vi "lv_buzzer.vi"() -> ()   [LabVIEW 2016]
panel:
  in  "Slide":dbl(slide) scale=0.0..10.0
  in  "Boolean 12":bool
  in  "Boolean 11":bool
  in  "Boolean 9":bool
  in  "Boolean 6":bool
  out "Numeric 4":dbl caption="Strange"
  out "Boolean 10":bool caption="Strange"
  out "text":string
  out "Boolean 8":bool
  out "Boolean 7":bool
  in  "file path (use dialog)":path
  in  "Boolean 5":bool
  in  "Boolean 4":bool
  out "Numeric 3":dbl caption="Down"
  out "Numeric 2":dbl caption="Up"
  out "Charm":dbl
  out "Boolean 3":bool caption="Down"
  out "Boolean 2":bool caption="Up"
  out "Boolean":bool caption="Charm"
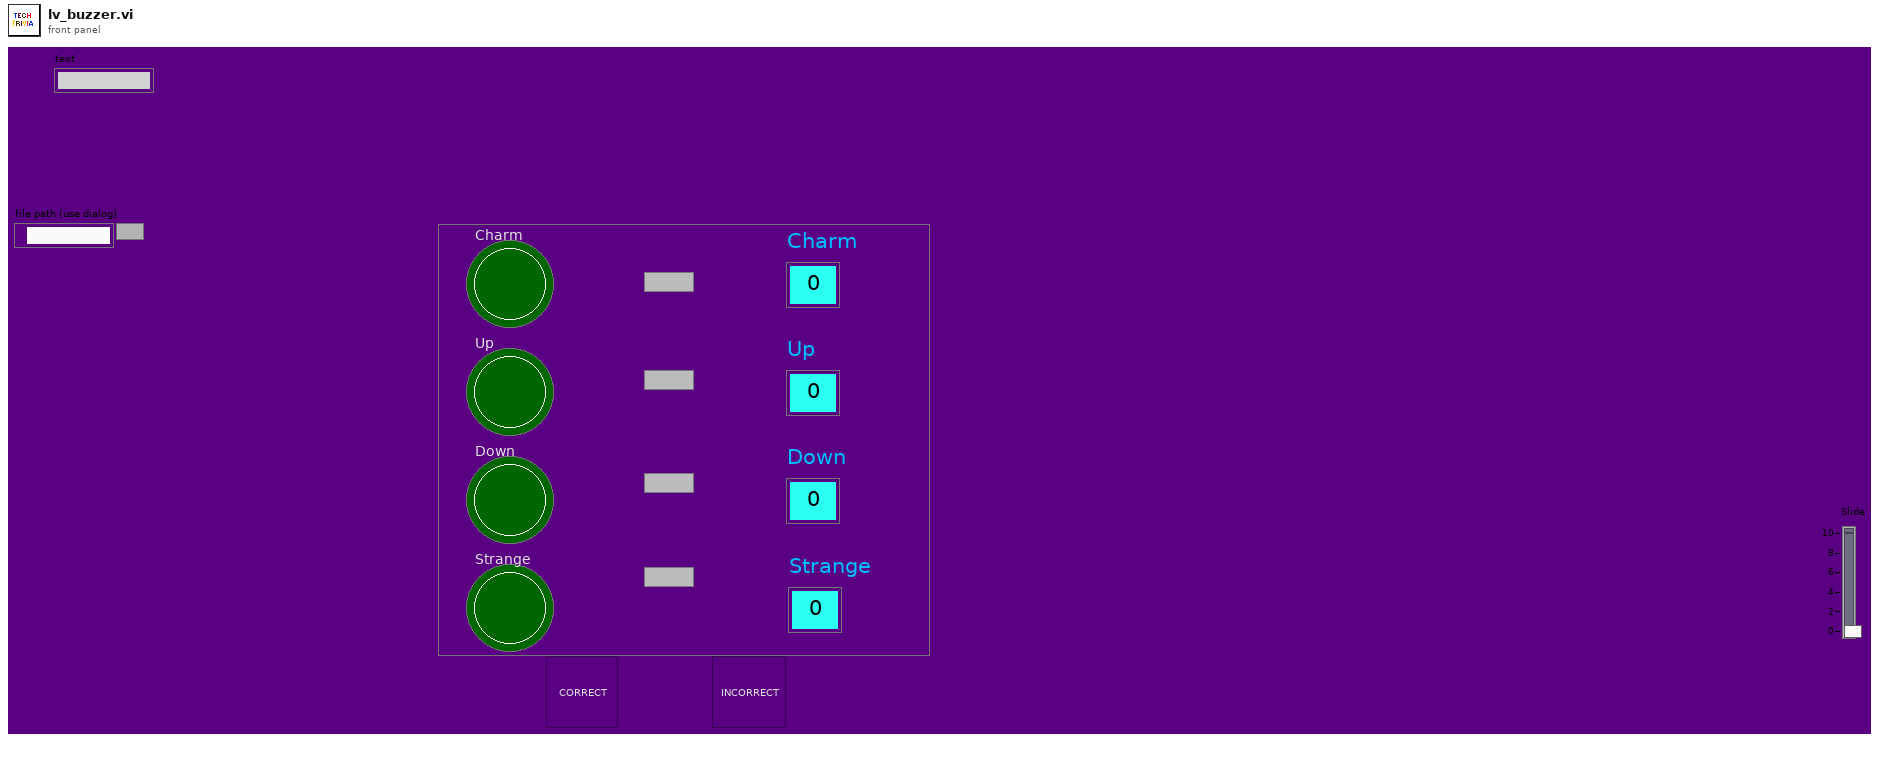
[diagram p1: front panel]
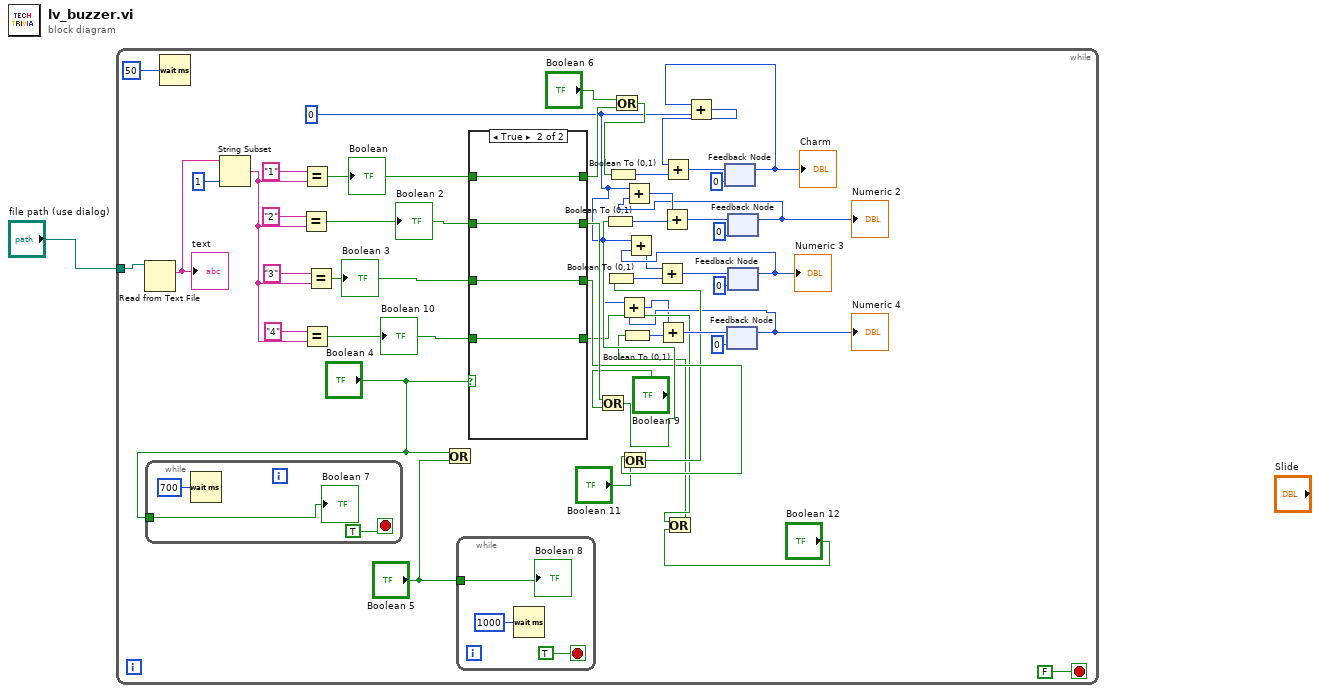
[diagram p0: block diagram]
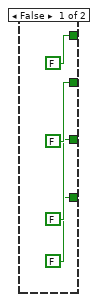
[diagram p2: hidden frame]
diagram:
  n1 = while {
    tunnel: "file path (use dialog)" -> [w32]
    stop <- FALSE stop-if-true
    w4 = i16 0 ("y")
    n2 = Read from Text File(file (use dialog)=w32) -> (text=w38:string)  [unwired: 3 in, 3 out]
    "text" <- w38
    n3 = while {
      tunnel: "Boolean 4" -> [w56]
      stop <- TRUE stop-if-true
      n4 = Wait (ms)(milliseconds to wait=u32 700) -> ()  [unwired: 1 out]
      "Boolean 7" <- w56
    }
    n5 = Wait (ms)(milliseconds to wait=u32 50) -> ()  [unwired: 1 out]
    n6 = String Subset(string=w38, length (rest)=1 ("length (rest)")) -> (substring=w28:string)  [unwired: 1 in]
    n7 = Equal?(x="2", y=w28) -> (x = y?=w30:bool)
    "Boolean 2" <- w30
    n8 = Equal?(x="1", y=w28) -> (x = y?=w31:bool)
    "Boolean" <- w31
    n9 = Equal?(x="4", y=w28) -> (x = y?=w26:bool)
    "Boolean 10" <- w26
    n10 = Equal?(x="3", y=w28) -> (x = y?=w29:bool)
    "Boolean 3" <- w29
    n11 = Or(x="Boolean 4", y="Boolean 5") -> ()  [unwired: 1 out]
    n12 = while {
      tunnel: "Boolean 5" -> [w53]
      stop <- TRUE stop-if-true
      n13 = Wait (ms)(milliseconds to wait=u32 1000) -> ()  [unwired: 1 out]
      "Boolean 8" <- w53
    }
    n14 = case shown="True" "Boolean 4" {
      tunnel: w29 -> [_ w64]
      tunnel: [FALSE w64] -> w16
      tunnel: w30 -> [_ w63]
      tunnel: [FALSE w63] -> w19
      tunnel: w31 -> [_ w62]
      tunnel: [FALSE w62] -> w21
      tunnel: w26 -> [_ w61]
      tunnel: [FALSE w61] -> w13
      frame False {
      }
      frame True {
      }
    }
    n15 = Or(x=w19, y="Boolean 9") -> (x .or. y?=w18:bool)
    n16 = Boolean To (0,1)(Boolean=w18) -> (0, 1=w46:i16)
    n17 = Or(x="Boolean 6", y=w21) -> (x .or. y?=w20:bool)
    n18 = Boolean To (0,1)(Boolean=w20) -> (0, 1=w45:i16)
    n19 = Or(x=w16, y="Boolean 11") -> (x .or. y?=w14:bool)
    n20 = Boolean To (0,1)(Boolean=w14) -> (0, 1=w47:i16)
    n21 = Or(x=w13, y="Boolean 12") -> (x .or. y?=w11:bool)
    n22 = Boolean To (0,1)(Boolean=w11) -> (0, 1=w23:i16)
    n23 = feedback #1(i16 0) -> (w10:i16)
    "Charm" <- w10
    n24 = Add(x=w10, y=w4) -> (x+y=w9:i16)
    n25 = Add(x=w9, y=w45) -> (x+y=w44:i16)
    n26 = feedback-in #1(w44) -> ()
    n27 = feedback #2(i16 0) -> (w3:i16)
    "Numeric 4" <- w3
    n28 = Add(x=w4, y=w3) -> (x+y=w2:i16)
    n29 = Add(x=w2, y=w23) -> (x+y=w25:i16)
    n30 = feedback-in #2(w25) -> ()
    n31 = feedback #3(i16 0) -> (w7:i16)
    "Numeric 2" <- w7
    n32 = Add(x=w4, y=w7) -> (x+y=w8:i16)
    n33 = Add(x=w8, y=w46) -> (x+y=w40:i16)
    n34 = feedback-in #3(w40) -> ()
    n35 = feedback #4(i16 0) -> (w6:i16)
    "Numeric 3" <- w6
    n36 = Add(x=w4, y=w6) -> (x+y=w5:i16)
    n37 = Add(x=w5, y=w47) -> (x+y=w42:i16)
    n38 = feedback-in #4(w42) -> ()
  }
